vi "P_sat_correlation.vi"(3 "Temperature[C]":dbl) -> (0 "formula":string, 1 "P Sat[Pa]":dbl)   [LabVIEW 2017]
uses:
  <vilib>/gmath/NI_Gmath.lvlib
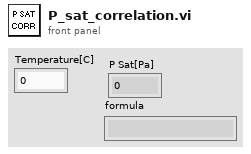
[diagram p1: front panel]
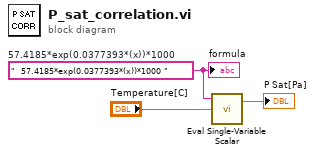
[diagram p0: block diagram]
diagram:
  w1 = "  57.4185*exp(0.0377393*(x))*1000 "  # 57.4185*exp(0.0377393*(x))*1000
  n1 = call <vilib>:"Eval Single-Variable Scalar.vi"("x value"="Temperature[C]", "formula"=w1) -> ("y value"=→"P Sat[Pa]":dbl)  [unwired: 1 in, 1 out]
  "formula" <- w1
